vi "英维克运行状态解析.vi"(11 "运行状态输入":u16[](array[numeric])) -> (3 "运行状态":T1)   [LabVIEW 2016, in "环境动力监测库.lvlib" / "空调库.lvlib"]
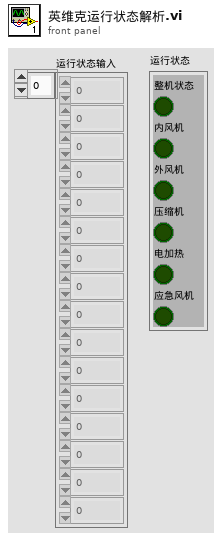
[diagram p1: front panel]
types:
  T1 = cluster{"整机状态":bool, "内风机":bool, "外风机":bool, "压缩机":bool, "电加热":bool, "应急风机":bool}
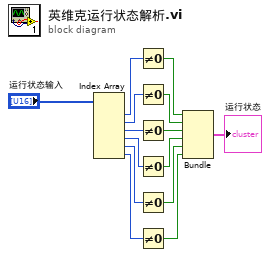
[diagram p0: block diagram]
diagram:
  n1 = Index Array(array="运行状态输入") -> (element #1=w13:u16, element #2=w12:u16, element #3=w11:u16, element #4=w10:u16, element #5=w9:u16, element #6=w8:u16)  [unwired: 6 in]
  n2 = Not Equal To 0?(x=w13) -> (x != 0?=w7:bool)
  n3 = Not Equal To 0?(x=w12) -> (x != 0?=w6:bool)
  n4 = Not Equal To 0?(x=w11) -> (x != 0?=w5:bool)
  n5 = Not Equal To 0?(x=w10) -> (x != 0?=w4:bool)
  n6 = Not Equal To 0?(x=w9) -> (x != 0?=w3:bool)
  n7 = Not Equal To 0?(x=w8) -> (x != 0?=w2:bool)
  n8 = Bundle(w7, w6, w5, w4, w3, w2) -> (→"运行状态":cluster{bool, bool, bool, bool, bool, bool})  [unwired: 1 in]
